vi "class_data.vi"() -> ()   [LabVIEW 2010, in "FPGAWrapperAN110607Galvo.lvclass"]
uses:
  FPGAWrapperAN110607Galvo.lvclass
  FPGA_VI_ref.ctl
panel:
  in  "FPGA VI reference":T1
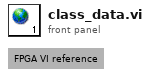
[diagram p1: front panel]
types:
  T1 = typedef "FPGAWrapperAN110607Galvo.lvclass/FPGA_VI_ref.ctl" = refnum<k20>
diagram:
